vi "Query Trigger Slope.vi"(8 "error in (no error)":errorcluster, 11 "VISA resource name":refnum<visa-resource-name>) -> (0 "error out":errorcluster, 2 "output":enum16{"Rise", "Fall"}(ring), 3 "VISA resource name out":refnum<visa-resource-name>)   [LabVIEW 2015, in "SR400.lvlib"]
doc: "TS { j }\nIf j = 1, the TS command sets the gate trigger\nslope to FALL or negative. If j = 0, the gate trigger\nslope is set to RISE or positive. If j is absent, the\ngate trigger slope is returned."
uses:
  SR400.lvlib
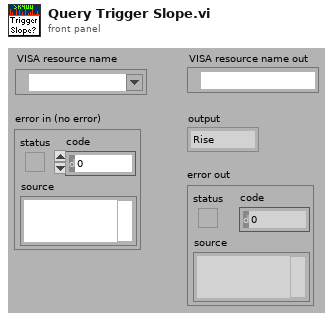
[diagram p1: front panel]
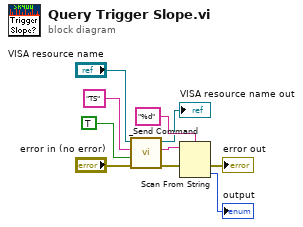
[diagram p0: block diagram]
diagram:
  n1 = call "_Send Command.vi"("error in (no error)"="error in (no error)", "Query? (F)"=TRUE, "Command"="TS" ("command"), "VISA resource name"="VISA resource name") -> ("error out"=w2:errorcluster, "Response"=w3:string, "VISA resource name out"=→"VISA resource name out":refnum<visa-resource-name>)  [unwired: 5 out]
  n2 = Scan From String(format string="%d", input string=w3, error in=w2) -> (error out=→"error out":errorcluster, output 1=→"output":enum16{"Rise", "Fall"})  [unwired: 1 in, 3 out]
